vi "Global Constants.vi"() -> ()   [LabVIEW 2014]
panel:
  in  "Header D":dbl
  in  "Header I":dbl
  in  "Header P":dbl
  in  "Robot Length":dbl=22.0
  in  "Robot Width":dbl=20.5
  in  "Resolver BR Low Voltage":dbl=0.196533
  in  "Resolver BR High Voltage":dbl=4.7229
  in  "Resolver BL Low Voltage":dbl=0.202637
  in  "Resolver BL High Voltage":dbl=4.70703
  in  "Resolver FR Low Voltage":dbl=0.203857
  in  "Resolver FR High Voltage":dbl=4.72778
  in  "Resolver FL Low Voltage":dbl=0.203857
  in  "Resolver FL High Voltage":dbl=4.7229
  in  "Example":dbl=-1.0
  in  "Offset BR":dbl=-1.0
  in  "Offset BL":dbl=-1.0
  in  "Offset FR":dbl=-1.0
  in  "Offset FL":dbl=-1.0
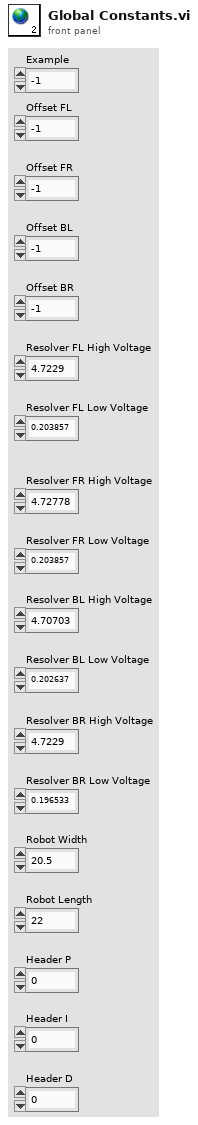
[diagram p1: front panel]
diagram:
